vi "lua_tostring.vi"(8 "error in (no error)":errorcluster, 10 "index":i32, 11 "lua_state_p":u64) -> (0 "error out":errorcluster, 2 "string":string, 3 "lua_state_p out":u64)   [LabVIEW 2020, in "lua.dll.lvlib"]
uses:
  lua.dll.lvlib
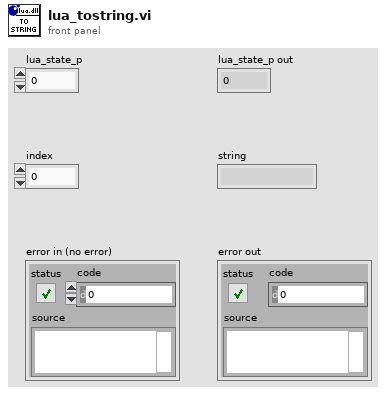
[diagram p1: front panel]
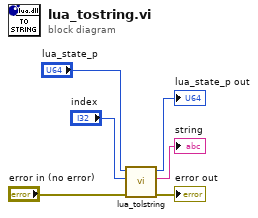
[diagram p0: block diagram]
diagram:
  n1 = call "lua_tolstring.vi"("error in (no error)"="error in (no error)", "index"="index", "lua_state_p"="lua_state_p") -> ("error out"=→"error out":errorcluster, "string"=→"string":string, "lua_state_p out"=→"lua_state_p out":u64)  [unwired: 6 in]
